vi "EnableCell.vi"(0 "DigitalCol in":refnum<class "DigitalCol.lvclass">, 5 "Cell Position":T1, 7 "Table Data in":string[][](array[string]), 9 "Table CtlRef In":refnum<vi>, 11 "error in (no error)":errorcluster) -> (4 "DigitalCol out":refnum<class "DigitalCol.lvclass">, 8 "Table Data out":string[][](array[string]), 10 "Table CtlRef Out":refnum<vi>, 15 "error out":errorcluster)   [LabVIEW 2013, in "DigitalCol.lvclass"]
uses:
  DigitalCol.lvclass
  <vilib>/Utility/miscctls.llb/LVRowAndColumnTypeDef.ctl
  Column/Column.lvclass/Column.ctl
  Column/Column.lvclass
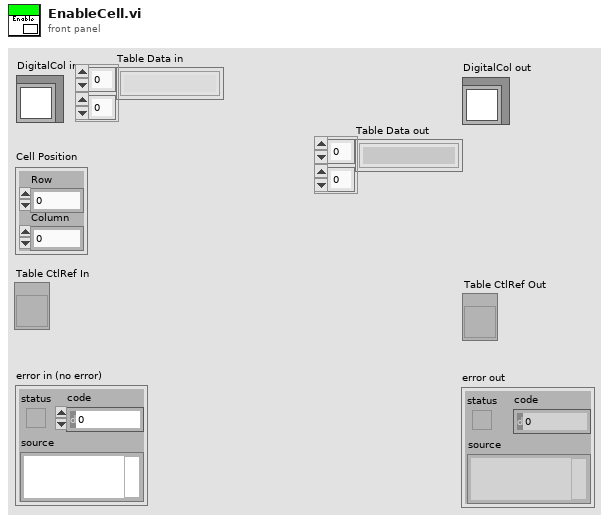
[diagram p1: front panel]
types:
  T1 = typedef "LVRowAndColumnTypeDef.ctl" = cluster{"Row":i32, "Column":i32}
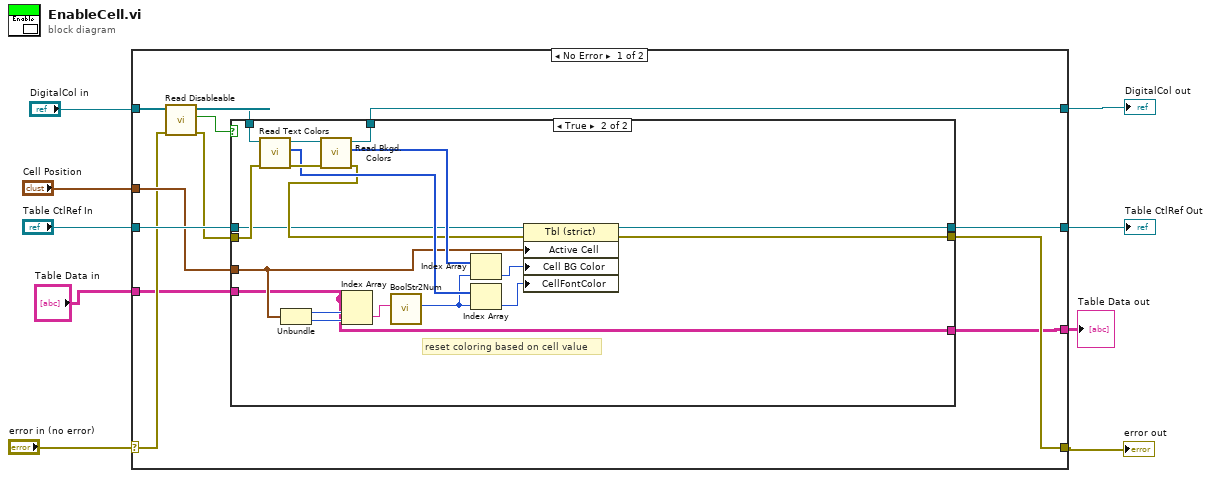
[diagram p0: block diagram]
diagram:
  n1 = case shown="No Error" "error in (no error)" {
    selector: "error in (no error)" -> [w14 w48]
    tunnel: [w18 w48] -> w9
    tunnel: [w12 w47] -> w7
    tunnel: "DigitalCol in" -> [w17 w47]
    tunnel: "Cell Position" -> [w19 _]
    tunnel: "Table CtlRef In" -> [w21 w46]
    tunnel: [w20 w46] -> w8
    tunnel: "Table Data in" -> [w11 w45]
    tunnel: [w10 w45] -> w1
    frame No Error {
      n2 = call "Read Disableable.vi"("error in (no error)"=w14, "Column in"=w17) -> ("error out"=w16:errorcluster, "Disableable?"=w15:bool, "Column out"=w13:refnum<class "DigitalCol.lvclass">)  [unwired: 7 in]
      n3 = case shown="True" w15 {
        tunnel: w21 -> [w25 w27]
        tunnel: [w25 w44] -> w20
        tunnel: w19 -> [_ w33]
        tunnel: w16 -> [w24 w37]
        tunnel: [w24 w43] -> w18
        tunnel: w13 -> [w23 w40]
        tunnel: [w23 w38] -> w12
        tunnel: w11 -> [w22 w26]
        tunnel: [w22 w26] -> w10
        frame False {
          # "Do nothing if column must always be enabled!"
        }
        frame True {
          # "reset coloring based on cell value"
          n4 = call "Read Text Colors.vi"("error in (no error)"=w37, "Column in"=w40) -> ("error out"=w36:errorcluster, "Text Colors"=w34:u32[], "Column out"=w39:refnum<class "DigitalCol.lvclass">)  [unwired: 7 in]
          n5 = Unbundle(w33) -> ("Row"=w32:i32, "Column"=w31:i32)
          n6 = call "Read Bkgd. Colors.vi"("error in (no error)"=w36, "Column in"=w39) -> ("error out"=w28:errorcluster, "Bkgd. Colors"=w35:u32[], "Column out"=w38:refnum<class "DigitalCol.lvclass">)  [unwired: 7 in]
          n7 = Index Array(array=w26, index (row)=w32, index (col)=w31) -> (element=w30:string)
          n8 = call "BoolStr2Num.vi"("Boolean string"=w30) -> ("number"=w29:i32)  [unwired: 10 in]
          n9 = Index Array(array=w35, index=w29) -> (element=w42:u32)
          n10 = Index Array(array=w34, index=w29) -> (element=w41:u32)
          n11 = property class="Tbl (strict)"(reference=w27, error in=w28, "Active Cell"=w33, "Cell BG Color"=w42, "CellFontColor"=w41) -> (reference out=w44:refnum<vi>, error out=w43:errorcluster)
        }
      }
    }
    frame Error {
    }
  }
  "error out" <- w9
  "DigitalCol out" <- w7
  "Table CtlRef Out" <- w8
  "Table Data out" <- w1
